vi "FPGA V3 torque test harness.vi"() -> ()   [LabVIEW 2018]
uses:
  <vilib>/ptbypt/NI_PtbyPt.lvlib
  <vilib>/Analysis/NI_AALBase.lvlib
panel:
  out "filteredState":bool
  in  "filter params":T1={"filterSize"=50, "lowerThreshold"=5, "upperThreshold"=45}
  in  "torque ripple":dbl format="%#_13g"
  in  "phase":dbl=250.0 format="%#_13g"
  out "S":u32
  out "Speed":sgl(graph)
  out "angle":u32 caption="angle (ticks)"
  out "speed":sgl caption="speed (rads/tick)"
  in  "amplitude":dbl=1.0 format="%#_13g"
  in  "speed (Hz)":dbl=666.0 format="%#_13g"
  in  "switch encoders":bool
  in  "rising edge (T)":bool
  in  "STOP":bool=TRUE
  out "Angle (rads)":sgl(graph)
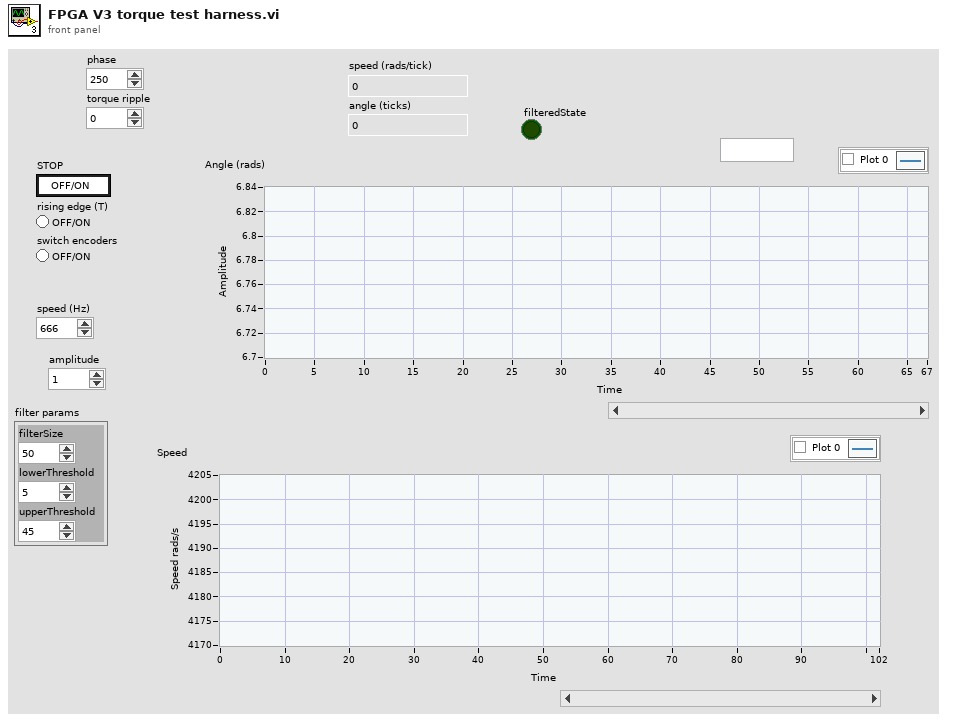
[diagram p1: front panel]
types:
  T1 = cluster{"filterSize":u8, "lowerThreshold":u8, "upperThreshold":u8}
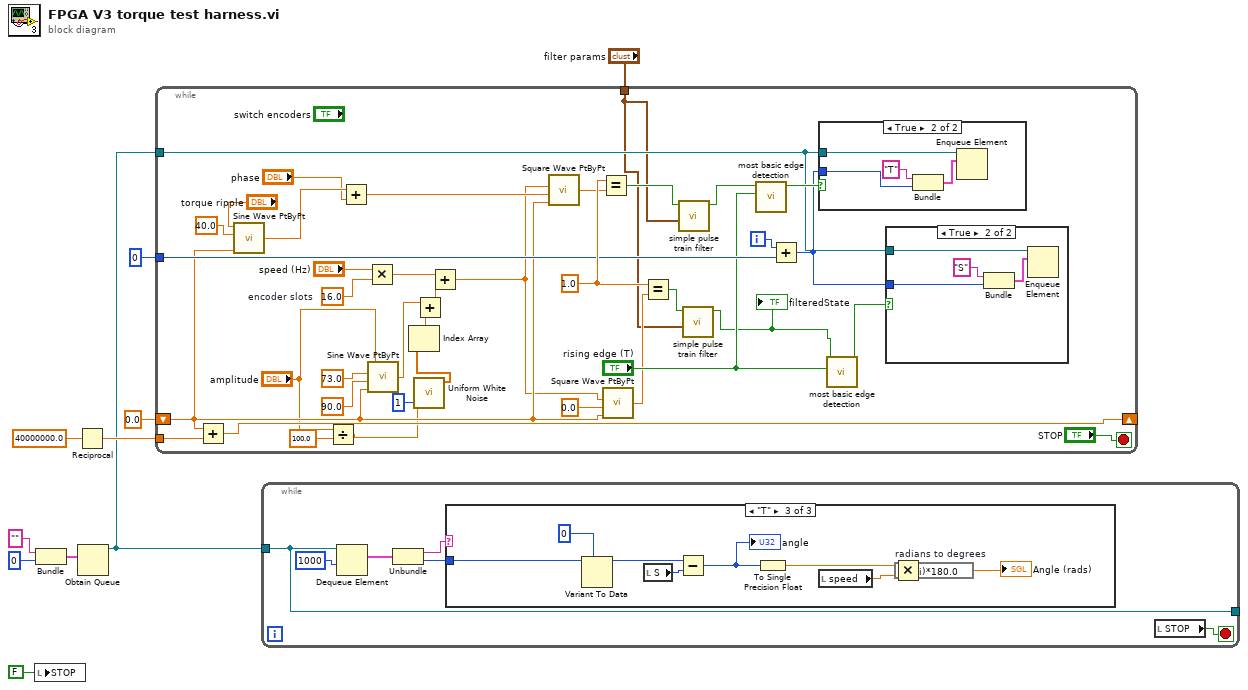
[diagram p0: block diagram]
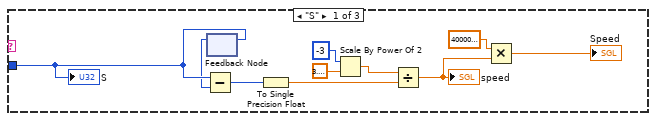
[diagram p2: hidden frame]
diagram:
  n1 = local write "STOP"(FALSE ("STOP")) -> ()
  n2 = Bundle("", "x+y"=u32 0) -> (w4:cluster{string, "x+y":u32})  [unwired: 1 in]
  n3 = Reciprocal(x=40000000.0 ("frequency")) -> (1/x=w9:dbl)
  n4 = Obtain Queue(element data type=w4) -> (queue out=w3:refnum<queue>)  [unwired: 4 in, 2 out]
  n5 = while {
    shift-right: [w47] -> _
    shift-left: 0.0 ("frequency") -> [w34]
    tunnel: w9 -> [w48]
    tunnel: u32 0 ("dimension size") -> [w39]
    tunnel: w3 -> [w25]
    tunnel: "filter params" -> [w11]
    i -> [w40]
    stop <- "STOP" stop-if-true
    w38 = 16.0  # encoder slots
    w46 = 1.0 ("x")
    n6 = Add(x=w34, y=w48) -> (x+y=w47:dbl)
    n7 = call <vilib>:"Sine Wave PtByPt.vi"("time"=w34, "frequency"=40.0, "amplitude"="torque ripple") -> ("sine wave"=w43:dbl)  [unwired: 1 in]
    n8 = Divide(x="amplitude", y=100.0) -> (x/y=w17:dbl)
    n9 = Add(x=w43, y="phase") -> (x+y=w41:dbl)
    n10 = Multiply(x="speed (Hz)", y=w38) -> (x*y=w37:dbl)
    n11 = call <vilib>:"Sine Wave PtByPt.vi"("time"=w34, "phase"=90.0, "frequency"=73.0, "amplitude"="amplitude") -> ("sine wave"=w20:dbl)
    n12 = call <vilib>:"Uniform White Noise.vi"("amplitude"=w17, "samples"=1) -> ("uniform white noise"=w23:dbl[])  [unwired: 8 in, 1 out]
    n13 = Index Array(array=w23) -> (element=w22:dbl)  [unwired: 1 in]
    n14 = Add(x=w20, y=w22) -> (x+y=w21:dbl)
    n15 = Add(x=w37, y=w21) -> (x+y=w33:dbl)
    n16 = call <vilib>:"Square Wave PtByPt.vi"("frequency"=w33, "phase"=w41, "time"=w34) -> ("square wave"=w31:dbl)  [unwired: 2 in]
    n17 = Equal?(x=w46, y=w31) -> (x = y?=w15:bool)
    n18 = call <vilib>:"Square Wave PtByPt.vi"("frequency"=w33, "phase"=0.0, "time"=w34) -> ("square wave"=w16:dbl)  [unwired: 2 in]
    n19 = Equal?(x=w46, y=w16) -> (x = y?=w13:bool)
    n20 = call "simple pulse train filter.vi"("filter params"=w11, "realState"=w15) -> ("filteredState"=w14:bool)  [unwired: 9 in]
    n21 = call "simple pulse train filter.vi"("filter params"=w11, "realState"=w13) -> ("filteredState"=w12:bool)  [unwired: 9 in]
    "filteredState" <- w12
    n22 = call "most basic edge detection.vi"("falling edge"="rising edge (T)", "pulse"=w14) -> ("edge detected"=w29:bool)  [unwired: 9 in]
    n23 = Add(x=w40, y=w39) -> (x+y=w26:u32)
    n24 = case shown="True" w29 {
      tunnel: w26 -> [_ w54]
      tunnel: w25 -> [_ w57]
      frame False {
      }
      frame True {
        n25 = Bundle("T", w54) -> (w56:cluster{string, u32})  [unwired: 1 in]
        n26 = Enqueue Element(queue=w57, element=w56) -> ()  [unwired: 2 in, 3 out]
      }
    }
    n27 = call "most basic edge detection.vi"("falling edge"="rising edge (T)", "pulse"=w12) -> ("edge detected"=w27:bool)  [unwired: 9 in]
    n28 = case shown="True" w27 {
      tunnel: w26 -> [_ w50]
      tunnel: w25 -> [_ w53]
      frame False {
      }
      frame True {
        n29 = Bundle("S", w50) -> (w52:cluster{string, u32})  [unwired: 1 in]
        n30 = Enqueue Element(queue=w53, element=w52) -> ()  [unwired: 2 in, 3 out]
      }
    }
  }
  n31 = while {
    tunnel: w3 -> [w59]
    tunnel: [w59] -> _
    stop <- w63 stop-if-true
    n32 = Dequeue Element(queue=w59, timeout in ms (-1)=1000) -> (element=w62:cluster{string, "x+y":u32})  [unwired: 1 in, 3 out]
    n33 = Unbundle(w62) -> (w61:string, "x+y"=w60:u32)
    n34 = case shown="\"T\"" w61 {
      tunnel: w60 -> [w68 _ w82]
      frame "S" {
        n35 = feedback #1() -> (w67:u32)  [unwired: 1 in]
        n36 = Subtract(x=w68, y=w67) -> (x-y=w70:u32)
        n37 = feedback-in #1(w68) -> ()
        n38 = To Single Precision Float(number=w70) -> (single precision float=w71:sgl)
        n39 = Scale By Power Of 2(n=i16 -3, x=sgl 3.1415927) -> (x*2^n=w64:sgl)
        n40 = Divide(x=w64, y=w71) -> (x/y=w72:sgl)
        "speed" <- w72
        n41 = Multiply(x=sgl 40000000.0, y=w72) -> (x*y=→"Speed":sgl)
        "S" <- w68
      }
      frame Default {
      }
      frame "T" {
        n42 = Variant To Data(type=u32 0 ("x+y"), Variant=w82) -> (data=w76:u32)  [unwired: 1 in, 1 out]
        n43 = local read "S"() -> (w75:u32)
        n44 = Subtract(x=w76, y=w75) -> (x-y=w77:u32)
        "angle" <- w77
        n45 = To Single Precision Float(number=w77) -> (single precision float=w79:sgl)
        n46 = local read "speed"() -> (w78:sgl)
        n47 = Multiply(x=w79, y=w78) -> (x*y=w80:sgl)
        n48 = expression code="(x/pi)*180.0" "radians to degrees"(w80) -> (→"Angle (rads)":sgl)
      }
    }
    n49 = local read "STOP"() -> (w63:bool)
  }
